vi "RFT Projekt  - Email küldése észleléskor -Design - Háttér szerkesztése.vi"() -> ()   [LabVIEW 2020]
uses:
  <vilib>/Instr/_visa.llb/VISA Configure Serial Port (Instr).vi
  <vilib>/smtpClient/Set Message Text.vi
  <vilib>/Utility/file.llb/Write Delimited Spreadsheet (string).vi
  <vilib>/smtpClient/LabVIEWSMTPClient.lvlib
panel:
  in  "Adatokat fogadó e-mail cím megadása":string
  in  "Csatolmány":path[](array[path])
  out "Feszültségérték: 2":string
  out "Aktuális idõ 2":string
  out "Mozgás érzékelve":bool
  in  "CSV Fájl mentési helye:":path
  in  "Port Kiválasztása":refnum<visa-resource-name>
  in  "Stop Button":bool
  # "Kommunikácós portok"
  # "Adatbázis"
  # "Levelezõ beállításai"
  # "V"
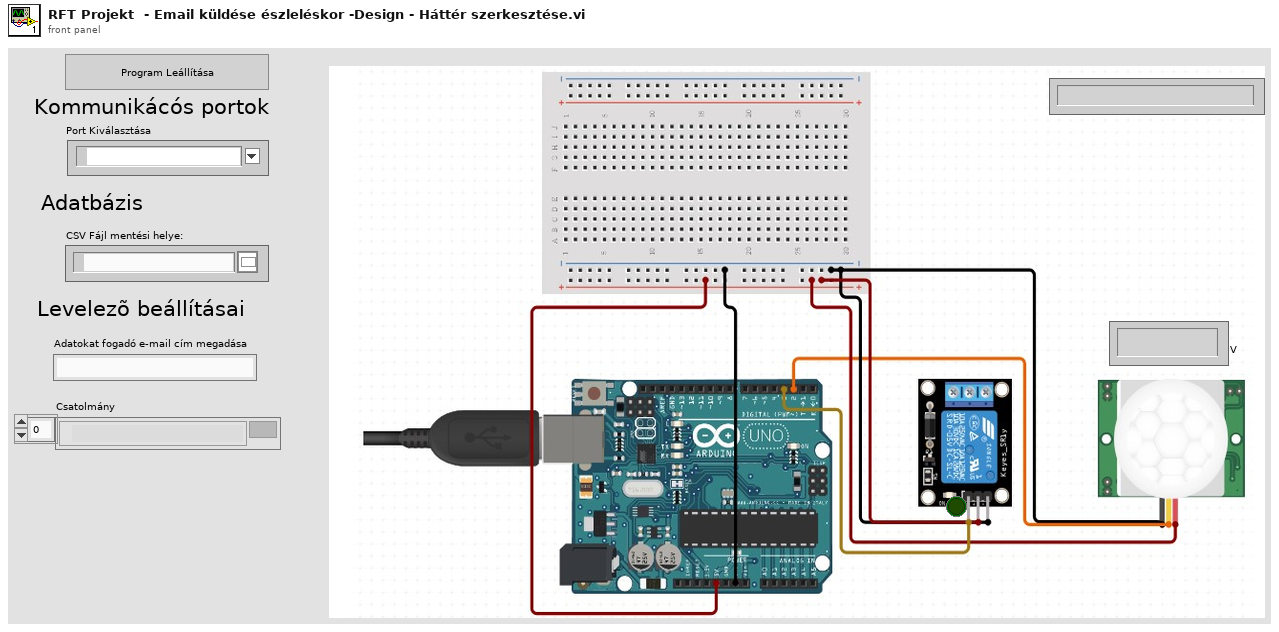
[diagram p1: front panel]
types:
  T1 = typedef "LabVIEWSMTPClient.lvlib/SmtpClientHandle.ctl" = refnum<k1>
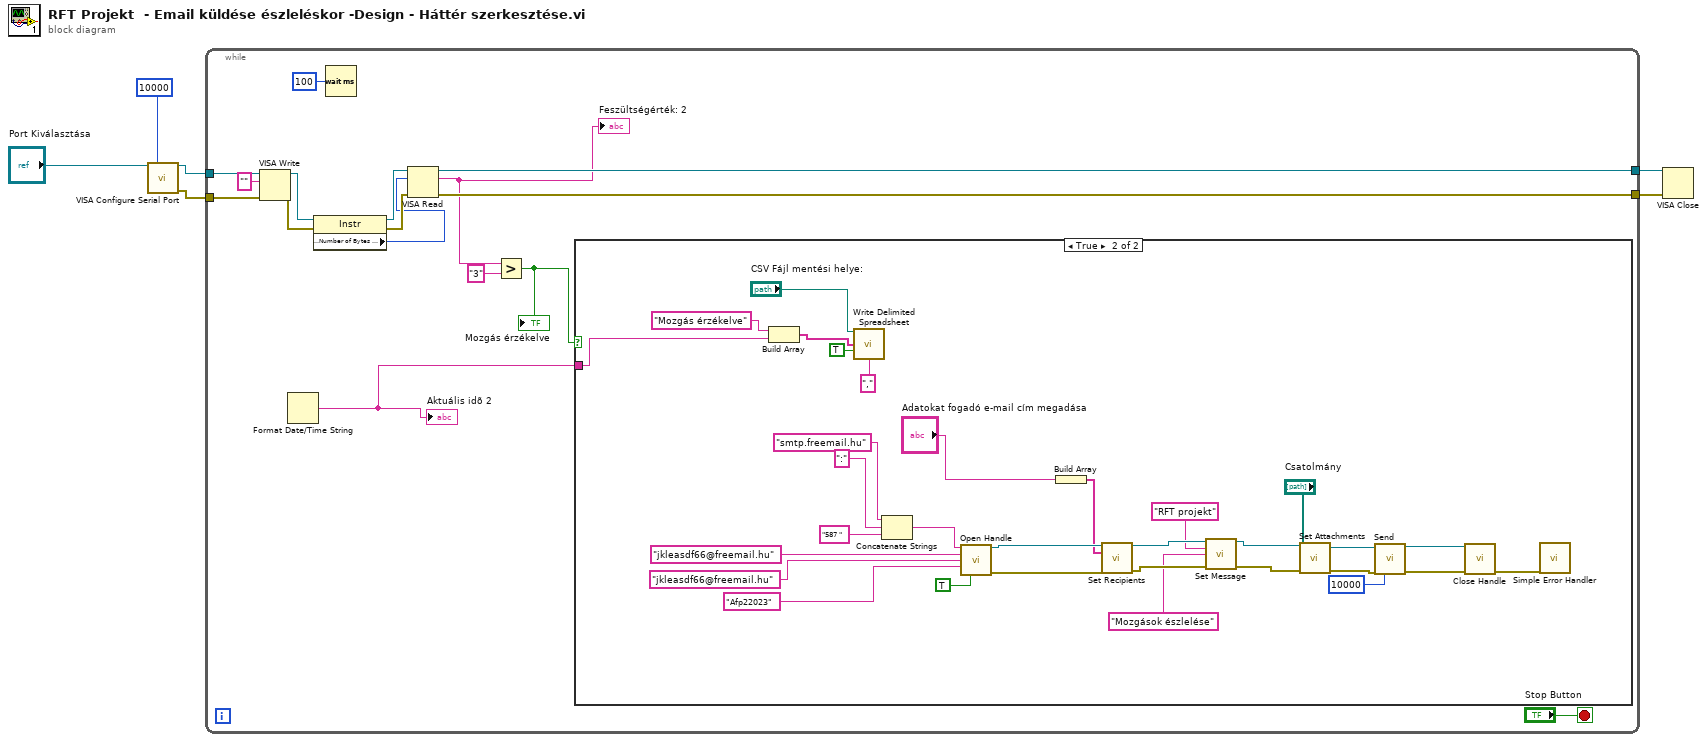
[diagram p0: block diagram]
diagram:
  n1 = call-poly "VISA Configure Serial Port"("VISA resource name"="Port Kiválasztása", "timeout (10sec)"=u32 10000) -> ("VISA resource name out"=w5:refnum<visa-resource-name>, "error out"=w3:errorcluster)  [unwired: 12 in]
  n2 = while {
    tunnel: w5 -> [w22]
    tunnel: [w21] -> w4
    tunnel: w3 -> [w20]
    tunnel: [w19] -> w2
    stop <- "Stop Button" stop-if-true
    n3 = VISA Write(VISA resource name=w22, write buffer="", error in (no error)=w20) -> (VISA resource name out=w18:refnum<visa-resource-name>, error out=w16:errorcluster)  [unwired: 1 out]
    n4 = Format Date/Time String() -> (date/time string=w8:string)  [unwired: 3 in]
    "Aktuális idõ 2" <- w8
    n5 = property class="Instr"(reference=w18, error in=w16) -> (reference out=w17:refnum<visa-resource-name>, error out=w15:errorcluster, "Serial Settings:Number of Bytes at Serial Port"=w14:u32)
    n6 = Wait (ms)(milliseconds to wait=u32 100) -> ()  [unwired: 1 out]
    n7 = VISA Read(VISA resource name=w17, byte count=w14, error in (no error)=w15) -> (VISA resource name out=w21:refnum<visa-resource-name>, read buffer=w7:string, error out=w19:errorcluster)  [unwired: 1 out]
    "Feszültségérték: 2" <- w7
    n8 = Greater?(x=w7, y="3") -> (0:w9:bool)
    "Mozgás érzékelve" <- w9
    n9 = case shown="True" w9 {
      tunnel: w8 -> [_ w50]
      frame False {
      }
      frame True {
        n10 = Build Array("Mozgás érzékelve", w50) -> (w49:string[])
        n11 = call-poly <vilib>:"Write Delimited Spreadsheet.vi"("file path (dialog if empty)"="CSV Fájl mentési helye:", "1D data"=w49, "append to file? (new file:F)"=TRUE, "delimiter (\\t)"="," ("delimiter (\\t)")) -> ()  [unwired: 10 in, 2 out]
        n12 = Concatenate Strings("smtp.freemail.hu" ("string"), ":" ("string"), "587 " ("string")) -> (w39:string)
        n13 = call <vilib>:"Open Handle.vi"("server address"=w39, "from"="jkleasdf66@freemail.hu" ("username"), "username"="jkleasdf66@freemail.hu", "password"="Afp22023", "use TLS (false)"=TRUE) -> ("handle out"=w36:T1, "error out"=w42:errorcluster)  [unwired: 9 in]
        n14 = Build Array("Adatokat fogadó e-mail cím megadása") -> (w23:string[])
        n15 = call <vilib>:"Set Recipients.vi"("handle in"=w36, "to"=w23, "error in (no error)"=w42) -> ("handle out"=w37:T1, "error out"=w43:errorcluster)  [unwired: 11 in]
        n16 = call-poly <vilib>:"Set Message.vi"("handle in"=w37, "subject"="RFT projekt", "plain text message"="Mozgások észlelése", "error in (no error)"=w43) -> ("handle out"=w40:T1, "error out"=w44:errorcluster)  [unwired: 10 in]
        n17 = call <vilib>:"Set Attachments.vi"("handle in"=w40, "attachments"="Csatolmány", "error in (no error)"=w44) -> ("handle out"=w41:T1, "error out"=w45:errorcluster)  [unwired: 11 in]
        n18 = call <vilib>:"Send.vi"("handle in"=w41, "error in (no error)"=w45, "timeout in ms (10000)"=10000) -> ("handle out"=w38:T1, "error out"=w46:errorcluster)  [unwired: 10 in, 1 out]
        n19 = call <vilib>:"Close Handle.vi"("handle in"=w38, "error in (no error)"=w46) -> ("error out"=w47:errorcluster)  [unwired: 12 in, 1 out]
        n20 = call <vilib>:"Simple Error Handler.vi"("error in (no error)"=w47) -> ()  [unwired: 4 in, 5 out]
      }
    }
  }
  n21 = VISA Close(VISA resource name=w4, error in (no error)=w2) -> ()  [unwired: 1 out]
